vi "PV Digiline relay switch point.vi"(8 "error in (no error)":errorcluster, 9 "DigiLine-Cluster":T1={"Parameter"=0, "Parameter\nread only<->describe"=FALSE, "Pressure switch point (mbar)"=1.0} {"Pressure switch point (mbar)" min=5e-10 max=2000.0 step=1.0 format="%_3e"; "Parameter" items=[" Pressure Set Point 1 [hPa ; mbar]", " Pressure Set Point 2 [hPa ; mbar]"]}, 10 "Adress of unit":u16=1 max=999 step=1, 11 "VISA session":refnum<visa-resource-name>) -> (0 "error out":errorcluster, 2 "response (data)":string, 3 "dup VISA session":refnum<visa-resource-name>)   [LabVIEW 2012, in "Pfeiffer Vacuum.lvlib"]
doc: "There are tow parameters available, only one of which can be enabled at a time. \n\n0 - Pressure switch point 1 [mbar] (default)\n1 - Pressure switch point 2 [mbar] \n\nNote: The one control right of this one will set the appropriate values for the selected parameter. Any settings for an parameter that is not selected will be ignored. If a value is out of range, it will be changed to either the upper or the lower limit of the range."
uses:
  <instrlib>/Pfeiffer Vacuum/Pfeiffer Vacuum.lvlib
  <instrlib>/Pfeiffer Vacuum/Public/DigiLine/Digiline relay switch point - Cluster.ctl
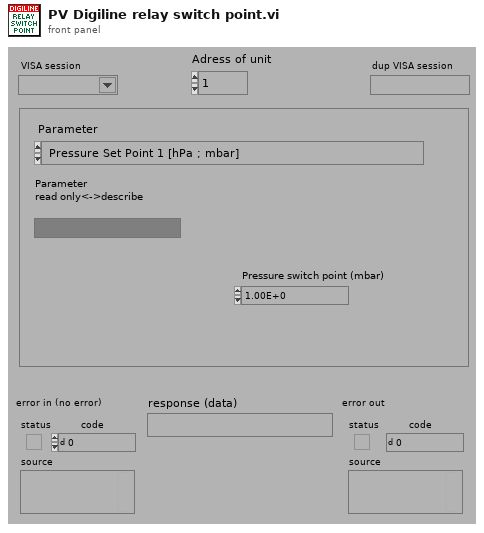
[diagram p1: front panel]
types:
  T1 = typedef "Pfeiffer Vacuum.lvlib/Digiline relay switch point - Cluster.ctl" = cluster{"Parameter":u16, "Parameter\nread only<->describe":bool, "Pressure switch point (mbar)":dbl}
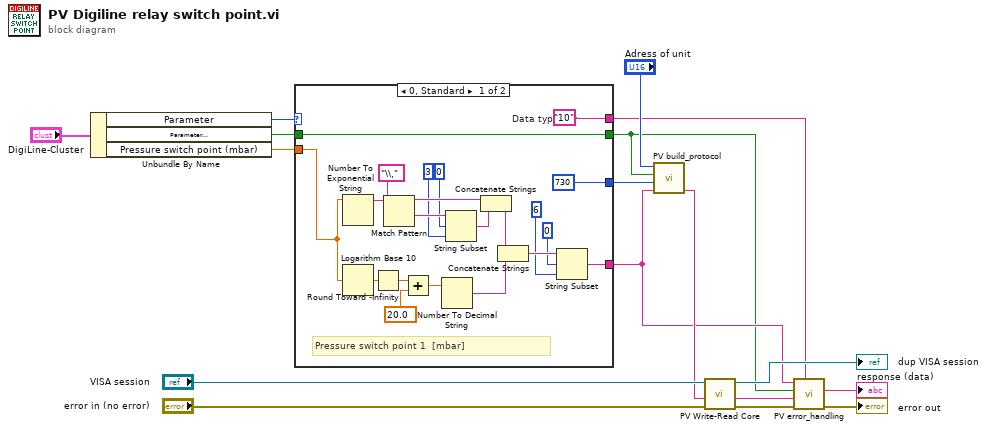
[diagram p0: block diagram]
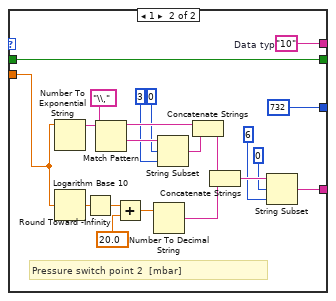
[diagram p2: hidden frame]
diagram:
  n1 = Unbundle By Name("DigiLine-Cluster") -> ("Parameter"=w14:u16, "Parameter\nread only<->describe"=w13:bool, "Pressure switch point (mbar)"=w1:dbl)
  n2 = case shown="0, Standard" w14 {
    tunnel: [u16 730 ("Parameter-number") u16 732 ("Parameter-number")] -> w16
    tunnel: [w18 w39] -> w4
    tunnel: [w37 w58] -> w3
    tunnel: w13 -> [w37 w58]
    tunnel: w1 -> [w19 w40]
    tunnel: [w36 w57] -> w5
    frame 0, Default {
      w36 = "10"  # Data typ
      # "Pressure switch point 1  [mbar]"
      n3 = Number To Exponential String(number=w19) -> (E-format string=w31:string)  [unwired: 3 in]
      n4 = Logarithm Base 10(1:w19) -> (0:w35:dbl)
      n5 = Round Toward -Infinity(1:w35) -> (0:w34:dbl)
      n6 = Match Pattern(string=w31, regular expression="\\,") -> (before substring=w32:string, after substring=w30:string)  [unwired: 1 in, 2 out]
      n7 = Add(x=w34, y=20.0) -> (x+y=w26:dbl)
      n8 = Number To Decimal String(number=w26) -> (decimal integer string=w23:string)  [unwired: 1 in]
      n9 = String Subset(string=w30, offset (0)=0 ("Offset (0)"), length (rest)=3 ("Länge")) -> (substring=w27:string)
      n10 = Concatenate Strings(w32, w27) -> (w24:string)
      n11 = Concatenate Strings(w24, w23) -> (w22:string)
      n12 = String Subset(string=w22, offset (0)=0 ("Offset (0)"), length (rest)=6 ("Länge")) -> (substring=w18:string)
    }
    frame 1 {
      w57 = "10"  # Data typ
      # "Pressure switch point 2  [mbar]"
      n13 = Number To Exponential String(number=w40) -> (E-format string=w52:string)  [unwired: 3 in]
      n14 = Logarithm Base 10(1:w40) -> (0:w56:dbl)
      n15 = Round Toward -Infinity(1:w56) -> (0:w55:dbl)
      n16 = Match Pattern(string=w52, regular expression="\\,") -> (before substring=w53:string, after substring=w51:string)  [unwired: 1 in, 2 out]
      n17 = Add(x=w55, y=20.0) -> (x+y=w47:dbl)
      n18 = Number To Decimal String(number=w47) -> (decimal integer string=w44:string)  [unwired: 1 in]
      n19 = String Subset(string=w51, offset (0)=0 ("Offset (0)"), length (rest)=3 ("Länge")) -> (substring=w48:string)
      n20 = Concatenate Strings(w53, w48) -> (w45:string)
      n21 = Concatenate Strings(w45, w44) -> (w43:string)
      n22 = String Subset(string=w43, offset (0)=0 ("Offset (0)"), length (rest)=6 ("Länge")) -> (substring=w39:string)
    }
  }
  n23 = call <instrlib>:"PV build_protocol.vi"("Data"=w4, "Parameter-number"=w16, "parameter\nread<->describe"=w3, "Adress"="Adress of unit") -> ("output"=w9:string)  [unwired: 3 in]
  n24 = call <instrlib>:"PV Write-Read Core.vi"("error in"="error in (no error)", "Write data in"=w9, "VISA session"="VISA session") -> ("error out"=w6:errorcluster, "response (data) out"=w7:string, "dup VISA session"=→"dup VISA session":refnum<visa-resource-name>)  [unwired: 2 in]
  n25 = call <instrlib>:"PV error_handling.vi"("Data Typ in"=w5, "error in"=w6, "response (data) in"=w7, "Parameter\nread only<->describe"=w3, "data in"=w4) -> ("error out"=→"error out":errorcluster, "Data out"=→"response (data)":string)  [unwired: 4 in, 1 out]
